vi "Tosca-Setup Pretrial Function.vi"(0 "Pretrial in":T1, 7 "Fs":dbl=50000.0) -> (4 "Pretrial out":T1, 8 "canceled":bool)   [LabVIEW 2020]
uses:
  Typedefs/Tosca-Pretrial Spec.ctl
  epl-vi-lib/Utility VIs/Controls/KPropertyTable/KPropertyTable.xctl
panel:
  in  "Path":path
  in  "Table":T2[](xcontrol)
  in  "Test":bool
  in  "Cancel":bool
  in  "OK":bool
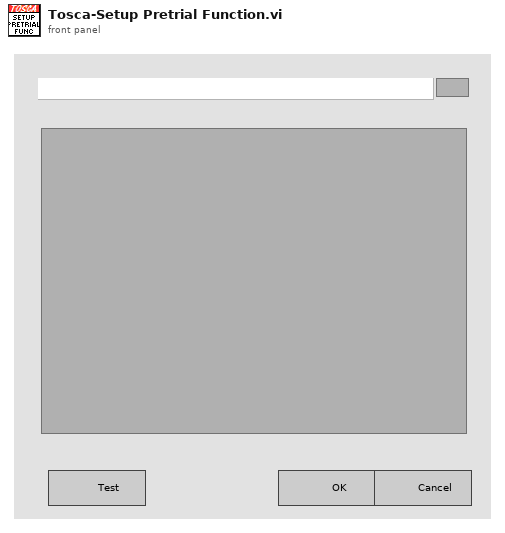
[diagram p1: front panel]
types:
  T1 = typedef "Tosca-Pretrial Spec.ctl" = cluster{"Path":path, "Args":string[]}
  T2 = typedef "KPropertyTable.xctl/RowData.ctl" = cluster{"Name":string, "Type":T3, "Category":string, "Strings":string[], "Value":string}
  T3 = typedef "KPropertyTable.xctl/DataType.ctl" = enum16{"String", "Enum", "Int", "Double", "Boolean", "Ring", "Formula"}
  T4 = enum8{"Enabled", "Disabled", "Disabled and Grayed Out"}
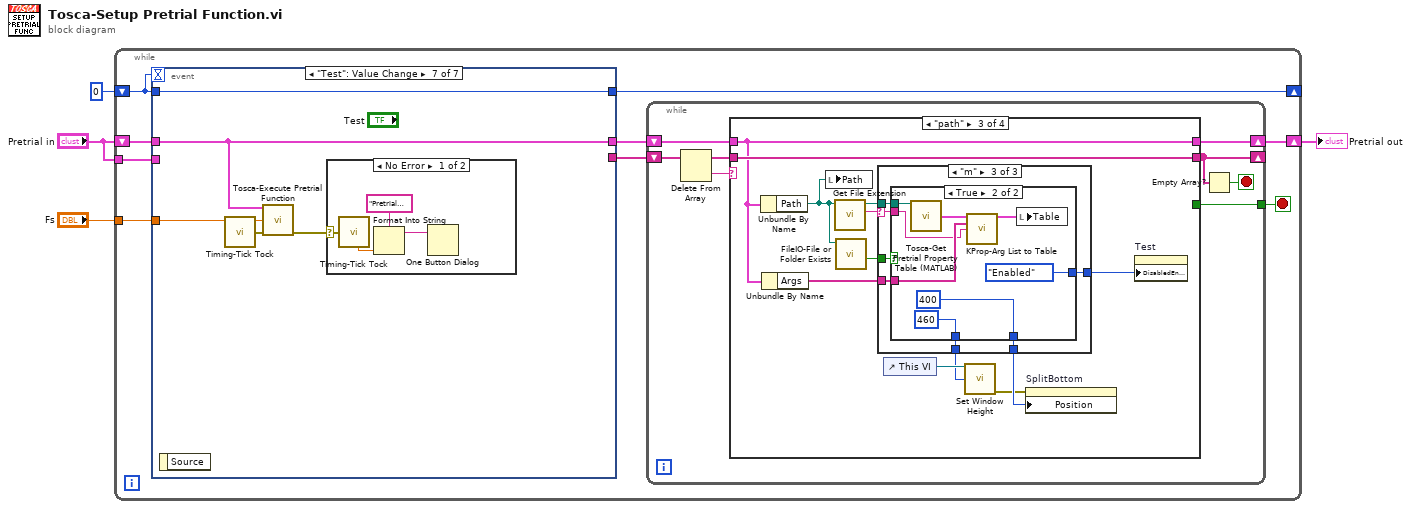
[diagram p0: block diagram]
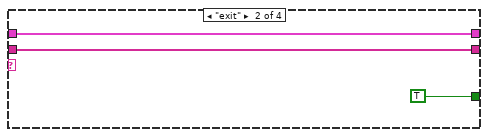
[diagram p3: hidden frame]
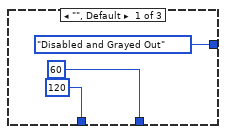
[diagram p4: hidden frame]
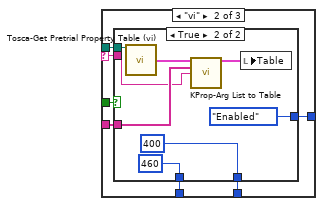
[diagram p5: hidden frame]
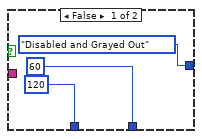
[diagram p6: hidden frame]
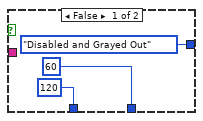
[diagram p7: hidden frame]
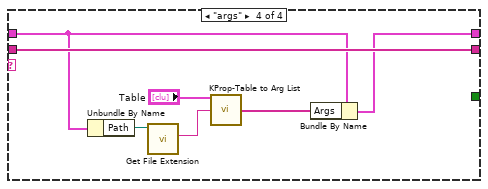
[diagram p8: hidden frame]
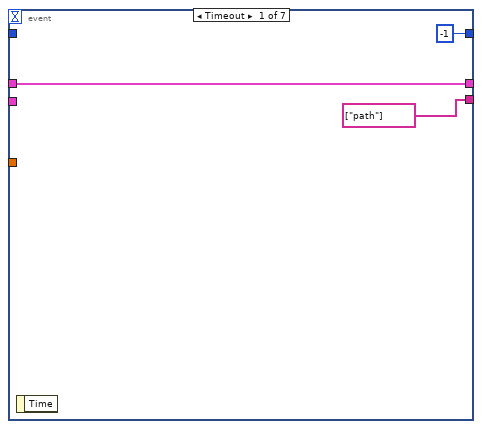
[diagram p9: hidden frame]
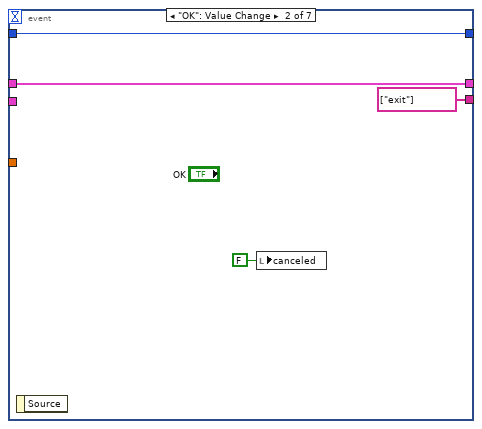
[diagram p10: hidden frame]
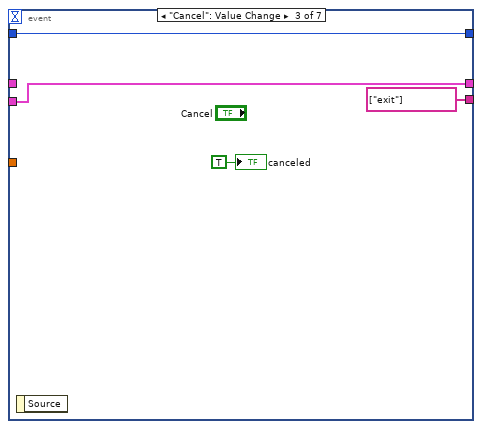
[diagram p11: hidden frame]
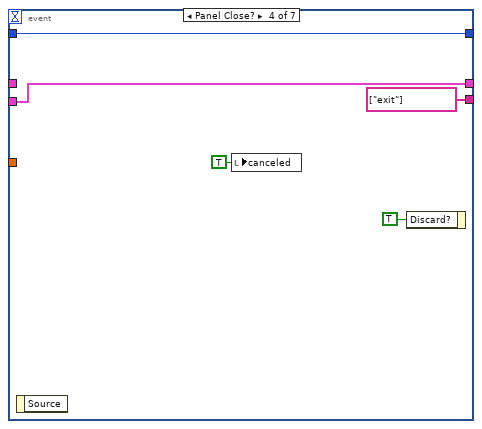
[diagram p12: hidden frame]
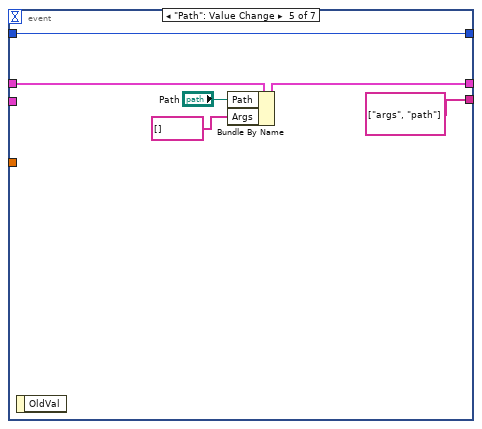
[diagram p13: hidden frame]
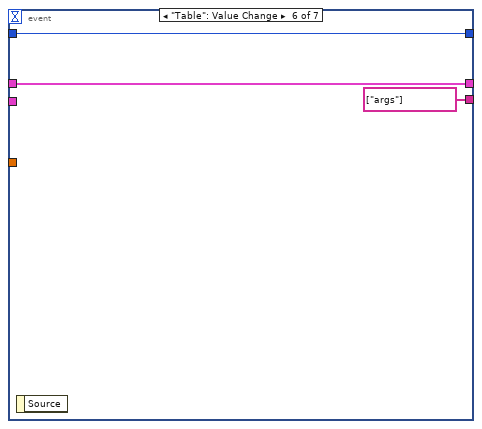
[diagram p14: hidden frame]
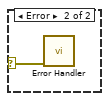
[diagram p15: hidden frame]
diagram:
  n1 = while {
    shift-right: [w8] -> w2
    shift-left: "Pretrial in" -> [w11]
    tunnel: "Pretrial in" -> [w6]
    shift-right: [w12] -> _
    shift-left: 0 -> [w13]
    tunnel: "Fs" -> [w5]
    stop <- w7 stop-if-true
    n2 = event shown="[6] \"Test\": Value Change" {
      selector: _ -> [_ _ _ _ _ _ _]
      dyn-events: _ -> [_ _ _ _ _ _ _]
      timeout: w13 -> [_ _ _ _ _ _ _]
      tunnel: w13 -> [_ w91 w95 w100 w106 w109 w114]
      tunnel: [-1 w91 w95 w100 w106 w109 w114] -> w12
      tunnel: w11 -> [w85 w90 _ _ w105 w108 w113]
      tunnel: [w85 w90 w94 w99 w104 w108 w113] -> w9
      tunnel: [string[] ["path"] string[] ["exit"] string[] ["exit"] string[] ["exit"] string[] ["args", "path"] string[] ["args"] _] -> w10
      tunnel: w6 -> [_ _ w94 w99 _ _ _]
      tunnel: w5 -> [_ _ _ _ _ _ w110]
      event Timeout {
        n3 = event-data() -> ()  [unwired: 1 in, 1 out]
      }
      event "OK": Value Change {
        n4 = event-data() -> ()  [unwired: 1 in, 1 out]
        n5 = local write "canceled"(FALSE ("canceled")) -> ()
      }
      event "Cancel": Value Change {
        n6 = event-data() -> ()  [unwired: 1 in, 1 out]
        "canceled" <- TRUE ("canceled")
      }
      event Panel Close? {
        n7 = event-data() -> ()  [unwired: 1 in, 1 out]
        n8 = local write "canceled"(TRUE ("canceled")) -> ()
        n9 = event-data("Discard?"=TRUE) -> ()  [unwired: 1 in, 1 out]
      }
      event "Path": Value Change {
        n10 = event-data() -> ()  [unwired: 1 in, 1 out]
        n11 = Bundle By Name(cluster=w105, "Path"="Path", "Args"=string[] []) -> (w104:T1)
      }
      event "Table": Value Change {
        n12 = event-data() -> ()  [unwired: 1 in, 1 out]
      }
      event "Test": Value Change {
        n13 = event-data() -> ()  [unwired: 1 in, 1 out]
        n14 = call "Timing-Tick Tock.vi"() -> ("error out"=w111:errorcluster)  [unwired: 6 in, 1 out]
        n15 = call "Tosca-Execute Pretrial Function.vi"("Pretrial in"=w113, "Fs"=w110, "error in (no error)"=w111) -> ("error out"=w112:errorcluster)  [unwired: 11 in, 1 out]
        n16 = case shown="No Error" w112 {
          selector: w112 -> [w118 w119]
          frame No Error {
            n17 = call "Timing-Tick Tock.vi"("error in (no error)"=w118) -> ("Elapsed time (ms)"=w117:dbl)  [unwired: 5 in, 1 out]
            n18 = Format Into String(format string="Pretrial function completed in %d ms.", w117) -> (resulting string=w115:string)  [unwired: 2 in, 1 out]
            n19 = One Button Dialog(message=w115) -> ()  [unwired: 1 in, 1 out]
          }
          frame Error {
            n20 = call "Error Handler.vi"("error in (no error)"=w119) -> ()  [unwired: 12 in, 3 out]
          }
        }
      }
    }
    n21 = while {
      shift-right: [w16] -> _
      shift-left: w10 -> [w21]
      shift-right: [w19] -> w8
      shift-left: w9 -> [w20]
      tunnel: [w14] -> w7
      stop <- w15 stop-if-true
      n22 = Delete From Array(array=w21) -> (deleted portion=w18:string, array with subset deleted=w17:string[])  [unwired: 2 in]
      n23 = case shown="\"path\"" w18 {
        tunnel: w20 -> [w23 w26 w32 w78]
        tunnel: [w23 w26 w32 w79] -> w19
        tunnel: w17 -> [w22 w25 w38 w84]
        tunnel: [w22 w25 w38 w84] -> w16
        tunnel: [_ TRUE _ _] -> w14
        frame "", Default {
        }
        frame "exit" {
        }
        frame "path" {
          n24 = Unbundle By Name(w32) -> ("Path"=w28:path)
          n25 = Unbundle By Name(w32) -> ("Args"=w30:string[])
          n26 = local write "Path"(w28) -> ()
          n27 = call <vilib>:"Get File Extension.vi"("file"=w28) -> ("lowercase file extension"=w37:string, "dup file"=w31:path)  [unwired: 6 in, 3 out]
          n28 = call "FileIO-File or Folder Exists.vi"("path"=w28) -> ("Exists?"=w27:bool)  [unwired: 7 in, 3 out]
          n29 = case shown="\"m\"" w37 {
            selector: w37 -> [_ w44 w62]
            tunnel: [60 w48 w66] -> w36
            tunnel: [120 w47 w65] -> w34
            tunnel: w31 -> [_ w46 w64]
            tunnel: w30 -> [_ w45 w63]
            tunnel: [T4."Disabled and Grayed Out" ("Disabled") w43 w61] -> w29
            tunnel: w27 -> [_ w42 w60]
            frame "", Default {
            }
            frame "vi" {
              n30 = case shown="True" w42 {
                tunnel: [60 400] -> w48
                tunnel: [120 460] -> w47
                tunnel: w46 -> [_ w57]
                tunnel: w45 -> [_ w54]
                tunnel: w44 -> [_ w53]
                tunnel: [T4."Disabled and Grayed Out" ("Disabled") T4."Enabled" ("Disabled")] -> w43
                frame False {
                }
                frame True {
                  n31 = call "Tosca-Get Pretrial Property Table (vi).vi"("Path"=w57) -> ("Table"=w56:T2[])  [unwired: 13 in, 1 out]
                  n32 = call "KProp-Arg List to Table.vi"("Rows in"=w56, "Args"=w54, "type"=w53) -> ("Rows out"=w55:T2[])  [unwired: 12 in]
                  n33 = local write "Table"(w55) -> ()
                }
              }
            }
            frame "m" {
              n34 = case shown="True" w60 {
                tunnel: [60 400] -> w66
                tunnel: [120 460] -> w65
                tunnel: w64 -> [_ w75]
                tunnel: w63 -> [_ w72]
                tunnel: w62 -> [_ w71]
                tunnel: [T4."Disabled and Grayed Out" ("Disabled") T4."Enabled" ("Disabled")] -> w61
                frame False {
                }
                frame True {
                  n35 = call "Tosca-Get Pretrial Property Table (MATLAB).vi"("Path"=w75) -> ("Table"=w74:T2[])  [unwired: 13 in, 1 out]
                  n36 = call "KProp-Arg List to Table.vi"("Rows in"=w74, "Args"=w72, "type"=w71) -> ("Rows out"=w73:T2[])  [unwired: 12 in]
                  n37 = local write "Table"(w73) -> ()
                }
              }
            }
          }
          n38 = control-ref of="This VI"() -> (w35:refnum<vi>)
          n39 = call "Set Window Height.vi"("VI in"=w35, "Height"=w34) -> ("error out"=w33:errorcluster)  [unwired: 12 in, 1 out]
          n40 = property on="SplitBottom" class="Splitter"(error in=w33, "Position"=w36) -> ()  [unwired: 1 in, 2 out]
          n41 = property on="Test" class="Bool"("DisabledEnum"=w29) -> ()  [unwired: 2 in, 2 out]
        }
        frame "args" {
          n42 = Unbundle By Name(w78) -> ("Path"=w80:path)
          n43 = call <vilib>:"Get File Extension.vi"("file"=w80) -> ("lowercase file extension"=w82:string)  [unwired: 6 in, 4 out]
          n44 = call "KProp-Table to Arg List.vi"("Rows"="Table", "type"=w82) -> ("Args"=w83:string[])  [unwired: 13 in]
          n45 = Bundle By Name(cluster=w78, "Args"=w83) -> (w79:T1)
        }
      }
      n46 = Empty Array?(array=w16) -> (empty?=w15:bool)
    }
  }
  "Pretrial out" <- w2
